vi "GdsLanguage_FindStrings.vi"(1 "SearchStringPattern":string, 5 "error in (no error)":errorcluster) -> (15 "StringsOut":string[](array[string]), 19 "error out":errorcluster)   [LabVIEW 2020]
doc: "Returns a translated string based on the value of the StringID parameter."
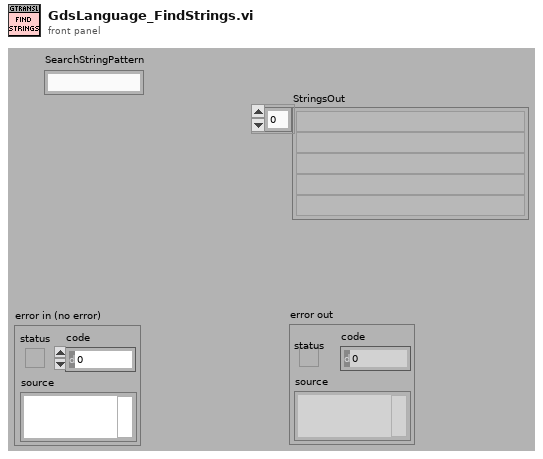
[diagram p1: front panel]
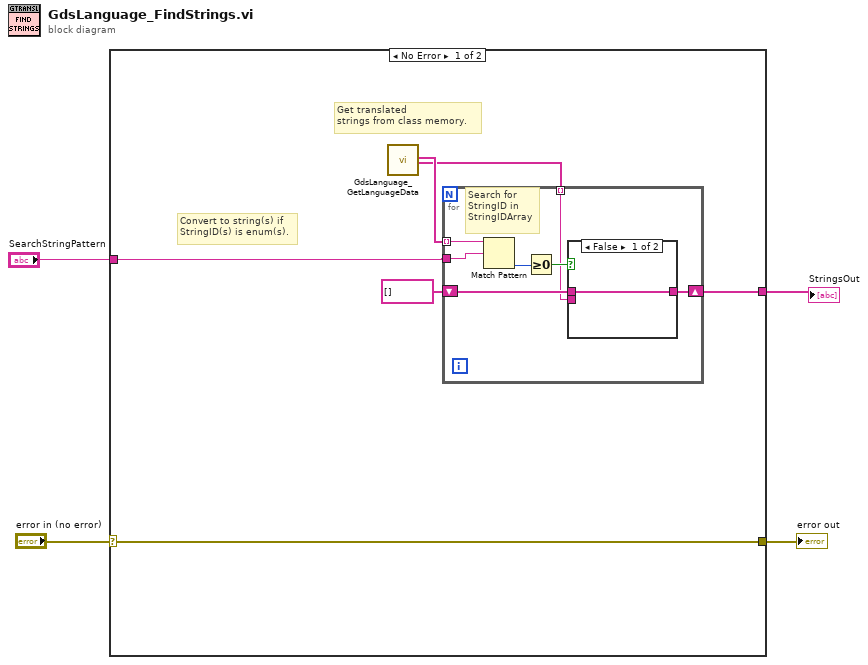
[diagram p0: block diagram]
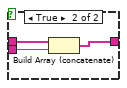
[diagram p2: hidden frame]
diagram:
  n1 = case shown="No Error" "error in (no error)" {
    selector: "error in (no error)" -> [w7 w22]
    tunnel: [w7 w22] -> w3
    tunnel: "SearchStringPattern" -> [w9 _]
    tunnel: [w8 _] -> w1
    frame No Error {
      # "Get translated\nstrings from class memory."
      # "Convert to string(s) if \nStringID(s) is enum(s)."
      n2 = call <resource>:"GdsLanguage_GetLanguageData.vi"() -> ("StringIDArray"=w10:string[], "TranslatedStrings"=w5:string[])  [unwired: 15 in, 3 out]
      n3 = for {
        tunnel: w9 -> [w17]
        tunnel: w10 -> [w13] mode=indexing
        shift-right: [w14] -> w8
        shift-left: string[] [] -> [w15]
        tunnel: w5 -> [w11] mode=indexing
        # "Search for\nStringID in \nStringIDArray"
        n4 = Match Pattern(string=w13, regular expression=w17) -> (offset past match=w16:i32)  [unwired: 1 in, 3 out]
        n5 = Greater Or Equal To 0?(x=w16) -> (x >= 0?=w12:bool)
        n6 = case shown="False" w12 {
          tunnel: w15 -> [w18 w21]
          tunnel: [w18 w20] -> w14
          tunnel: w11 -> [_ w19]
          frame False {
          }
          frame True {
            n7 = Build Array (concatenate)(w21, w19) -> (w20:string[])
          }
        }
      }
    }
    frame Error {
    }
  }
  "error out" <- w3
  "StringsOut" <- w1
